vi "Send Data to Waterfall for Octave.vi"(4 "settings":T2={"clear graph before redrawing (F)"=FALSE, "set baseline (F)"=FALSE, "baseline"=0.0, "autoscale (T)"=TRUE} {"baseline" format="%.2f"}, 5 "frontmost (T)":bool=TRUE, 6 "y0 and delta y":cluster{"y0":dbl, "delta y":dbl}={"y0"=0.0, "delta y"=1.0} {"delta y" format="%.2f"; "y0" format="%.2f"}, 7 "bandedge frequencies [Hz]":T1(array[cluster]) {"midband" format="%.2f"; "f high" format="%.2f"; "f low" format="%.2f"}, 8 "waterfall data":dbl[][](array[numeric]) format="%.2f", 9 "waterfall ref":refnum<vi>) -> (3 "dup waterfall ref":refnum<vi>)   [LabVIEW 2017]
doc: "Sends the waterfall data (octave spectra) to the waterfall display for octave. Use the settings cluster to specify how to display the new data."
uses:
  <vilib>/addons/Sound and Vibration/compatibility/Waterfall/subVIs/sv_Waterfall for Octave Global.vi
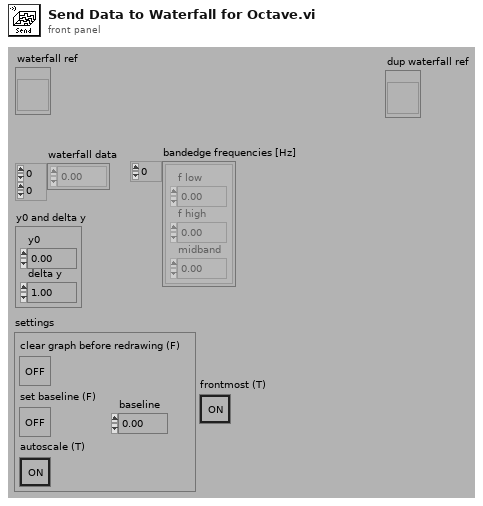
[diagram p1: front panel]
types:
  T1 = cluster{"f low":dbl, "f high":dbl, "midband":dbl}[]
  T2 = cluster{"clear graph before redrawing (F)":bool, "set baseline (F)":bool, "baseline":dbl, "autoscale (T)":bool}
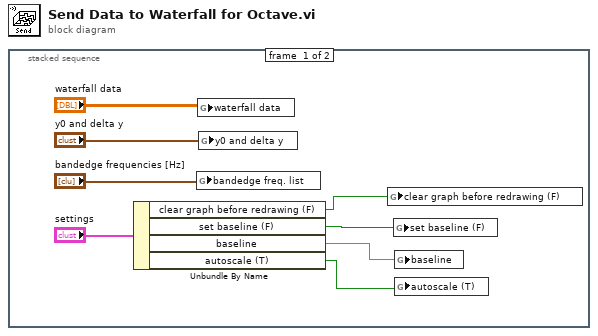
[diagram p0: block diagram]
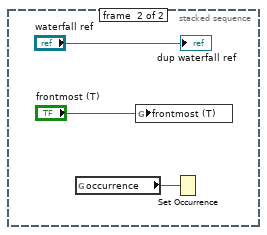
[diagram p2: hidden frame]
diagram:
  n1 = stacked-sequence {
    frame #0 {
      n2 = Unbundle By Name("settings") -> ("clear graph before redrawing (F)"=w5:bool, "set baseline (F)"=w4:bool, "baseline"=w3:dbl, "autoscale (T)"=w2:bool)
      n3 = global write "sv_Waterfall for Octave Global.vi" "bandedge freq. list"("bandedge frequencies [Hz]") -> ()
      n4 = global write "sv_Waterfall for Octave Global.vi" "waterfall data"("waterfall data") -> ()
      n5 = global write "sv_Waterfall for Octave Global.vi" "y0 and delta y"("y0 and delta y") -> ()
      n6 = global write "sv_Waterfall for Octave Global.vi" "clear graph before redrawing (F)"(w5) -> ()
      n7 = global write "sv_Waterfall for Octave Global.vi" "set baseline (F)"(w4) -> ()
      n8 = global write "sv_Waterfall for Octave Global.vi" "baseline"(w3) -> ()
      n9 = global write "sv_Waterfall for Octave Global.vi" "autoscale (T)"(w2) -> ()
    }
    frame #1 {
      n10 = global read "sv_Waterfall for Octave Global.vi" "occurrence"() -> (w11:refnum<k4>)
      n11 = global write "sv_Waterfall for Octave Global.vi" "frontmost (T)"("frontmost (T)") -> ()
      n12 = Set Occurrence(w11) -> ()
      "dup waterfall ref" <- "waterfall ref"
    }
  }
